vi "Read Data Titles.vi"(8 "error in (no error)":errorcluster, 11 "KeithleyMeter in":refnum<class "KeithleyMeter.lvclass">) -> (0 "error out":errorcluster, 2 "Data titles":string[](array[string])=["Signal"], 3 "KeithleyMeter out":refnum<class "KeithleyMeter.lvclass">)   [LabVIEW 2015, in "KeithleyMeter.lvclass"]
uses:
  KeithleyMeter.lvclass
  KeithleyMeter.lvclass/KeithleyMeter.ctl
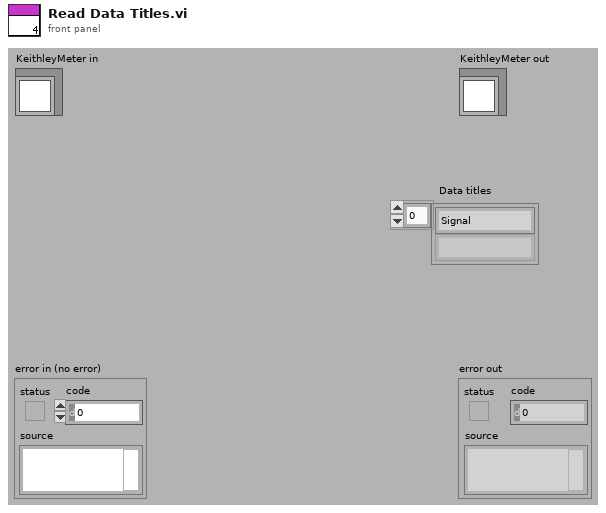
[diagram p1: front panel]
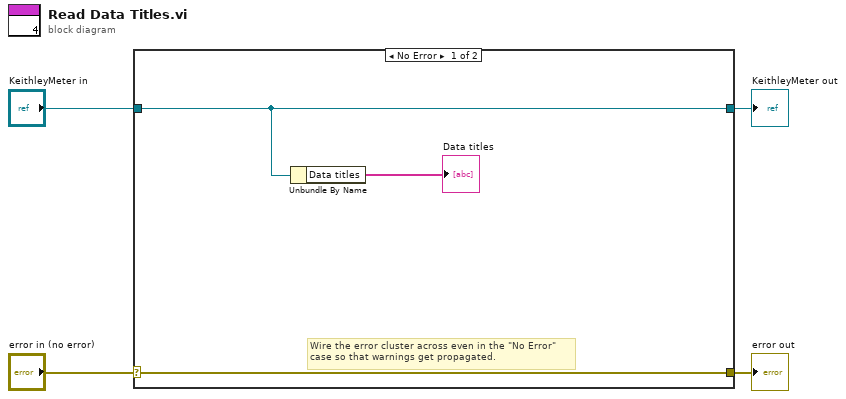
[diagram p0: block diagram]
diagram:
  n1 = case shown="No Error" "error in (no error)" {
    selector: "error in (no error)" -> [w7 w9]
    tunnel: [w7 w9] -> w3
    tunnel: [w6 w8] -> w1
    tunnel: "KeithleyMeter in" -> [w6 w8]
    frame No Error {
      # "Wire the error cluster across even in the \"No Error\"\ncase so that warnings get propagated."
      n2 = Unbundle By Name(w6) -> ("Data titles"=→"Data titles":string[])
    }
    frame Error {
    }
  }
  "error out" <- w3
  "KeithleyMeter out" <- w1
